vi "Netburner_cntlTCP.vi"(0 "Phase Volt":dbl=6.500000000000002 min=-9.0 max=9.0 step=0.0005 format="%_5f", 1 "Tune Volt":dbl=0.3670000000000009 min=-9.9 max=9.9 step=0.0005 format="%_5g", 3 "# Data":i32=80 min=1 max=500 step=1, 5 "IF Atten (dB)":i8=3 min=0 max=31 step=1, 7 "NMR ADC":i32 min=0 max=3 step=1, 8 "Hi Gain":bool, 9 "Tank RF":bool, 11 "LogOff Volt":dbl=-5.996000000000003 min=0.0 max=9.0 step=0.0005 format="%_5f", 12 "IFOff Volt":dbl=5.450461000000012 min=-9.9 max=9.9 step=0.0005 format="%_4g", 14 "# f steps":i32=81 min=1 max=1000 step=1) -> (2 "Temp (C)":dbl=26.88 format="%#_5g", 4 "ADC value":dbl[](array[numeric])=[-0.0314, -0.0313, -0.0297, -0.0295, -0.0285, -0.0272, -0.026, -0.0257, -0.0236, -0.0229, -0.0227, -0.0232, -0.0213, -0.0193, -0.0187, -0.018, -0.0166, -0.0148, -0.0136, -0.0136, -0.0124, -0.0123, -0.0121, -0.0127, -0.0131, -0.0123, -0.0127, -0.0125, -0.0133, -0.0128, -0.0117, -0.012, -0.0128, -0.0138, -0.0149, -0.0166, -0.0211, -0.0291, -0.0424, -0.043, -0.0352, -0.0325, -0.0302, -0.0273, -0.0269, -0.0277, -0.026, -0.0263, -0.0242, -0.021, -0.0178, -0.0171, -0.0172, -0.0168, -0.0161, -0.0168, -0.0178, -0.0197, -0.0204, -0.0197, -0.0175, -0.0187, -0.0188, -0.0202, -0.0207, -0.0229, -0.0238, -0.0251, -0.0264, -0.0268, -0.0278, -0.0301, -0.0313, -0.0334, -0.0364, -0.0377, -0.0382, -0.0394, -0.043, -0.0442, -0.0438], 6 "ADC Std Dev":dbl=0.0009679012345679012 format="%#_4g", 10 "Max ADC":dbl=-0.0117 format="%#_5g", 13 "Volts":dbl=3.245 format="%#_5g", 15 "Min ADC":dbl=-0.0442 format="%#_5g")   [LabVIEW 2018]
uses:
  Global 2.vi
  <vilib>/Analysis/NI_AALBase.lvlib
panel:
  out "Spill":dbl=3.245 format="%#_5g"
  out "ADC Voltage Chart":dbl(graph)=-0.0438
  out "Mean ADC":dbl=-0.023260493827160496 format="%#_5g"
  out "ADC result string":string=" 6.5000  0.3670 -5.9960  5.4505 0 80 81 6 0 0\r26.88  3.245  \r\n-0.0314 0.0005  \r\n-0.0313 0.0007  \r\n-0.0297 0.0008  \r\n-0.0295 0.0007  \r\n-0.0285 0.0009  \r\n-0.0272 0.0007  \r\n-0.0260 0.0009  \r\n-0.0257 0.0007  \r\n-0.0236 0.0008  \r\n-0.0229 0.0008  \r\n-0.0227 0.0009  \r\n-0.0232 0.0011  \r\n-0.0213 0.0010  \r\n-0.0193 0.0014  \r\n-0.0187 0.0009  \r\n-0.0180 0.0007  \r\n-0.0166 0.0010  \r\n-0.0148 0.0006  \r\n-0.0136 0.0007  \r\n-0.0136 0.0010  \r\n-0.0124 0.0006  \r\n-0.0123 0.0007  \r\n-0.0121 0.0007  \r\n-0.0127 0.0006  \r\n-0.0131 0.0006  \r\n-0.0123 0.0007  \r\n-0.0127 0.0007  \r\n-0.0125 0.0006  \r\n-0.0133 0.0006  \r\n-0.0128 0.0009  \r\n-0.0117 0.0006  \r\n-0.0120 0.0008  \r\n-0.0128 0.0006  \r\n-0.0138 0.0007  \r\n-0.0149 0.0009  \r\n-0.0166 0.0016  \r\n-0.0211 0.0031  \r\n-0.0291 0.0059  \r\n-0.0424 0.0009  \r\n-0.0430 0.0037  \r\n-0.0352 0.0010  \r\n-0.0325 0.0013  \r\n-0.0302 0.0016  \r\n-0.0273 0.0006  \r\n-0.0269 0.0007  \r\n-0.0277 0.0007  \r\n-0.0260 0.0009  \r\n-0.0263 0.0015  \r\n-0.0242 0.0014  \r\n-0.0210 0.0013  \r\n-0.0178 0.0010  \r\n-0.0171 0.0007  \r\n-0.0172 0.0007  \r\n-0.0168 0.0007  \r\n-0.0161 0.0006  \r\n-0.0168 0.0005  \r\n-0.0178 0.0010  \r\n-0.0197 0.0008  \r\n-0.0204 0.0010  \r\n-0.0197 0.0006  \r\n-0.0175 0.0006  \r\n-0.0187 0.0006  \r\n-0.0188 0.0010  \r\n-0.0202 0.0007  \r\n-0.0207 0.0006  \r\n-0.0229 0.0008  \r\n-0.0238 0.0009  \r\n-0.0251 0.0009  \r\n-0.0264 0.0008  \r\n-0.0268 0.0009  \r\n-0.0278 0.0008  \r\n-0.0301 0.0007  \r\n-0.0313 0.0006  \r\n-0.0334 0.0012  \r\n-0.0364 0.0009  \r\n-0.0377 0.0006  \r\n-0.0382 0.0007  \r\n-0.0394 0.0013  \r\n-0.0430 0.0012  \r\n-0.0442 0.0008  \r\n-0.0438 0.0009  \r\n?\r\n"
  out "DAC, ADC String":string=" 6.5000  0.3670 -5.9960  5.4505 0 80 81 6 0 0"
  out "Error Out":errorcluster={"status"=FALSE, "code"=1073676294, "source"="VISA Read in Netburner_RD.vi->Netburner_cntl6.vi"}
  # "Netburner ADC/DAC Test Interface, TCP I/O"
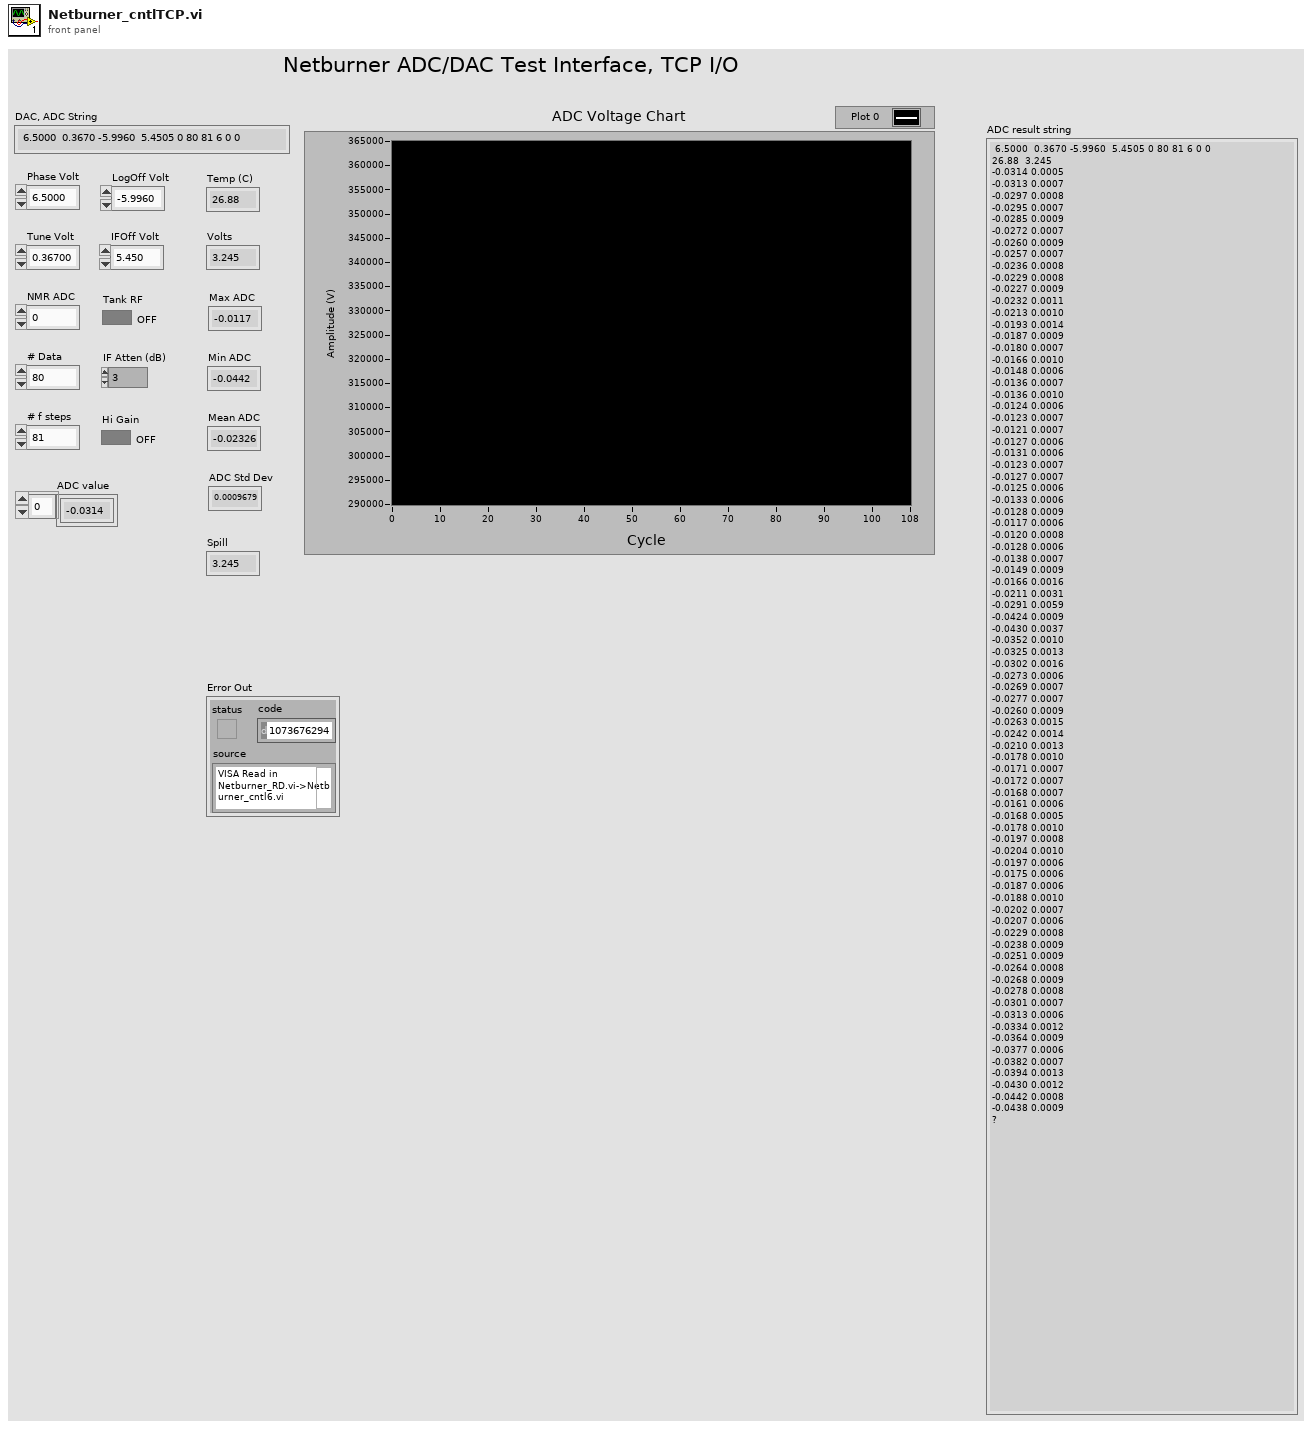
[diagram p1: front panel]
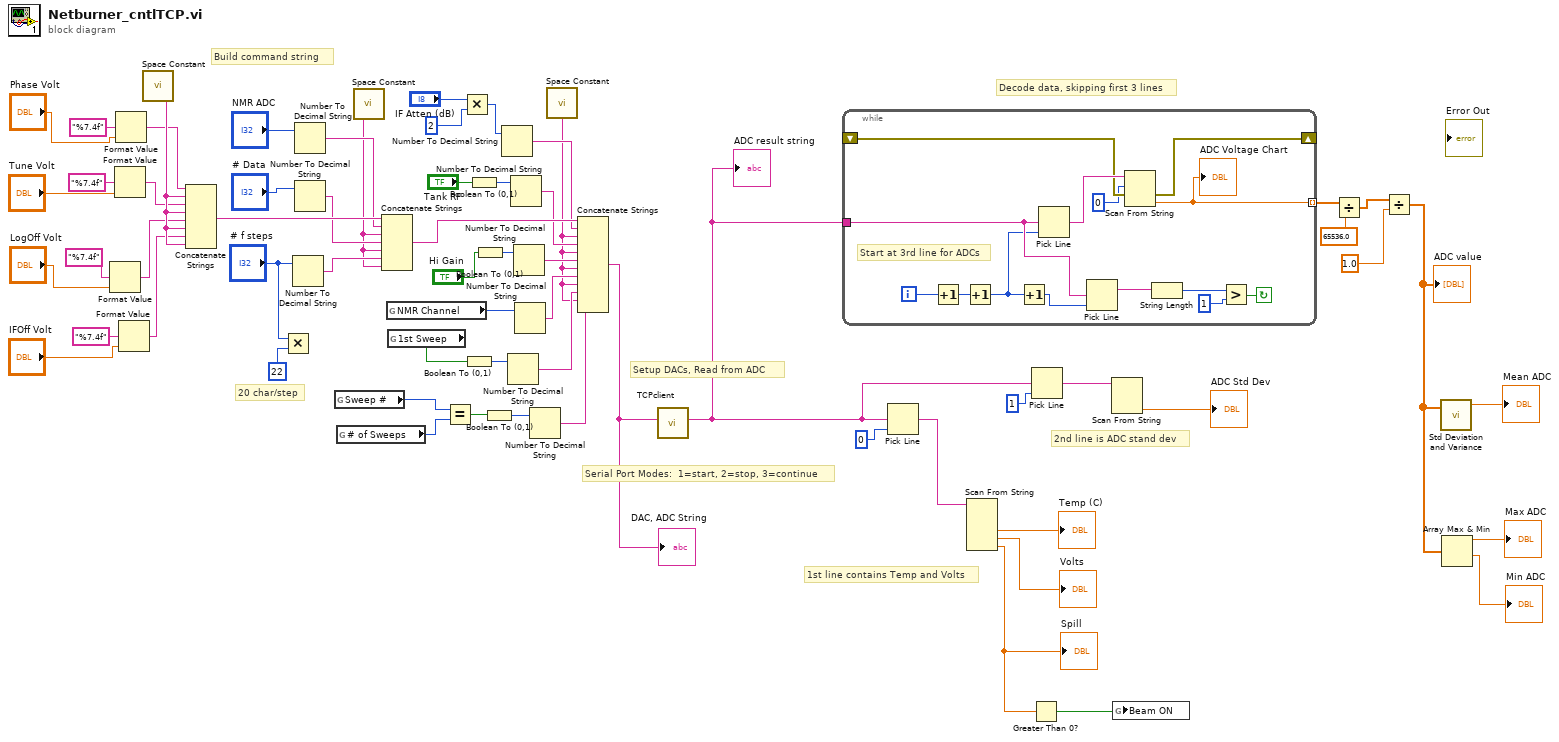
[diagram p0: block diagram]
diagram:
  # "2nd line is ADC stand dev"
  # "20 char/step"
  # "1st line contains Temp and Volts"
  # "Build command string"
  # "Decode data, skipping first 3 lines"
  # "Serial Port Modes:  1=start, 2=stop, 3=continue"
  # "Setup DACs, Read from ADC"
  n1 = Format Value(format string="%7.4f", value (0)="LogOff Volt") -> (output string=w24:string)  [unwired: 1 in]
  n2 = Format Value(format string="%7.4f", value (0)="Tune Volt") -> (output string=w48:string)  [unwired: 1 in]
  n3 = Format Value(format string="%7.4f", value (0)="Phase Volt") -> (output string=w26:string)  [unwired: 1 in]
  n4 = Format Value(format string="%7.4f", value (0)="IFOff Volt") -> (output string=w51:string)  [unwired: 1 in]
  n5 = call <vilib>:"Space Constant.vi"() -> ("String"=w57:string)
  n6 = Concatenate Strings(w26, w57, w48, w57, w24, w57, w51, w57) -> (w58:string)
  n7 = Multiply(x="# f steps", y=22) -> ()  [unwired: 1 out]
  n8 = Number To Decimal String(number="# f steps") -> (decimal integer string=w54:string)  [unwired: 1 in]
  n9 = Number To Decimal String(number="NMR ADC") -> (decimal integer string=w56:string)  [unwired: 1 in]
  n10 = Number To Decimal String(number="# Data") -> (decimal integer string=w55:string)  [unwired: 1 in]
  n11 = global read "Global 2.vi" "Sweep #"() -> (w11:i32)
  n12 = global read "Global 2.vi" "# of Sweeps"() -> (w10:i32)
  n13 = call <vilib>:"Space Constant.vi"() -> ("String"=w46:string)
  n14 = Concatenate Strings(w58, w56, w46, w55, w46, w54, w46) -> (w47:string)
  n15 = global read "Global 2.vi" "NMR Channel"() -> (w18:i32)
  n16 = global read "Global 2.vi" "1st Sweep"() -> (w14:bool)
  n17 = Equal?(x=w11, y=w10) -> (x = y?=w9:bool)
  n18 = Multiply(x="IF Atten (dB)", y=2) -> (x*y=w36:i32)
  n19 = Boolean To (0,1)(Boolean=w14) -> (0, 1=w13:i16)
  n20 = Boolean To (0,1)(Boolean="Tank RF") -> (0, 1=w44:i16)
  n21 = Boolean To (0,1)(Boolean="Hi Gain") -> (0, 1=w43:i16)
  n22 = Boolean To (0,1)(Boolean=w9) -> (0, 1=w6:i16)
  n23 = Number To Decimal String(number=w36) -> (decimal integer string=w45:string)  [unwired: 1 in]
  n24 = Number To Decimal String(number=w13) -> (decimal integer string=w12:string)  [unwired: 1 in]
  n25 = Number To Decimal String(number=w44) -> (decimal integer string=w42:string)  [unwired: 1 in]
  n26 = Number To Decimal String(number=w43) -> (decimal integer string=w41:string)  [unwired: 1 in]
  n27 = Number To Decimal String(number=w18) -> (decimal integer string=w17:string)  [unwired: 1 in]
  n28 = Number To Decimal String(number=w6) -> (decimal integer string=w7:string)  [unwired: 1 in]
  n29 = call <vilib>:"Space Constant.vi"() -> ("String"=w8:string)
  n30 = Concatenate Strings(w47, w45, w8, w42, w8, w41, w8, w17, w8, w12, w8, w7) -> (w20:string)
  "DAC, ADC String" <- w20
  n31 = call "TCPclient.vi"("Input Command"=w20) -> ("Command and Results"=w19:string)  [unwired: 3 in, 3 out]
  "ADC result string" <- w19
  n32 = while {
    tunnel: w19 -> [w75]
    tunnel: [w73] -> w5 mode=indexing
    shift-right: [w68] -> _
    shift-left: _ -> [w69]
    i -> [w65]
    stop <- w72 continue-if-true
    # "Start at 3rd line for ADCs"
    n33 = Increment(x=w65) -> (x+1=w66:i32)
    n34 = Increment(x=w66) -> (x+1=w64:i32)
    n35 = Increment(x=w64) -> (x+1=w76:i32)
    n36 = Pick Line(multi-line string=w75, line index=w64) -> (output string=w77:string)  [unwired: 1 in]
    n37 = Pick Line(multi-line string=w75, line index=w76) -> (output string=w74:string)  [unwired: 1 in]
    n38 = Scan From String "Scan From String"(input string=w77, initial scan location=0, error in=w69) -> (error out=w68:errorcluster, output 1=w73:dbl)  [unwired: 2 in, 2 out]
    "ADC Voltage Chart" <- w73
    n39 = String Length(string=w74) -> (length=w71:i32)
    n40 = Greater?(x=w71, y=1) -> (0:w72:bool)
  }
  n41 = Pick Line(multi-line string=w19, line index=0) -> (output string=w34:string)  [unwired: 1 in]
  n42 = Scan From String "Scan From String"(input string=w34) -> (output 1=→"Temp (C)":dbl, output 2=→"Volts":dbl, output 3=w16:dbl)  [unwired: 6 in, 3 out]
  "Spill" <- w16
  n43 = Greater Than 0?(x=w16) -> (x > 0?=w15:bool)
  n44 = Pick Line(multi-line string=w19, line index=1) -> (output string=w22:string)  [unwired: 1 in]
  n45 = Scan From String "Scan From String"(input string=w22) -> (output 1=→"ADC Std Dev":dbl)  [unwired: 4 in, 3 out]
  n46 = global write "Global 2.vi" "Beam ON"(w15) -> ()
  n47 = Divide(x=w5, y=65536.0) -> (x/y=w3:dbl[])
  n48 = Divide(x=w3, y=1.0) -> (x/y=w2:dbl[])
  "ADC value" <- w2
  n49 = call <vilib>:"Std Deviation and Variance.vi"("X"=w2) -> ("mean"=→"Mean ADC":dbl)  [unwired: 1 in, 2 out]
  n50 = Array Max & Min(array=w2) -> (max value=→"Max ADC":dbl, min value=→"Min ADC":dbl)  [unwired: 2 out]
